vi "IMAQdx Acquisition Template (Host).vi"() -> ()   [LabVIEW 2016]
uses:
  <vilib>/userdefined/High Color/IMAQdx.ctl
  <vilib>/vision/driver/IMAQdx.llb/IMAQdx Acquisition Mode.ctl
  <vilib>/vision/driver/IMAQdx.llb/IMAQdx Buffer Number Mode.ctl
  <vilib>/FPGAPlugInAG/roboRIO/niLvFpga_Open_roboRIO.vi
  <vilib>/rvi/interface/common/dynamic/niFpgaDynamicAddResources.vi
  <vilib>/FPGAPlugInAG/Dynamic/niLvFpga_Download_Dynamic.vi
  <vilib>/FPGAPlugInAG/Dynamic/niLvFpga_Run_Dynamic.vi
  <vilib>/visionFPGA/Basics/Configure Image Transfer to Target/IMAQ FPGA Configure Image Transfer to Target U32.vi
  <vilib>/Utility/error.llb/Error Cluster From Error Code.vi
  <vilib>/rvi/errors/niLvFpgaAdjustHostInterfaceError.vi
  <vilib>/visionFPGA/Basics/Image Transfer to Target/IMAQ FPGA Image Transfer to Target U32.vi
  <vilib>/rvi/interface/common/niFpgaWaitOnOcc.vi
  <vilib>/FPGAPlugInAG/Dynamic/niLvFpga_Close_Dynamic.vi
  <vilib>/rvi/interface/nirviOpenFPGA/nirviOpenFPGA.xnode
  FPGA Bitfiles/ImageProcessingw_FPGATarget2_ImageProcessingw_ZcF2hsHpmf8.lvbitx
  Image Processing with Vision Assistant (FPGA).vi
  <vilib>/rvi/interface/nirviMethod/nirviMethod.xnode
  <vilib>/rvi/interface/nirviReadWriteControl/nirviReadWriteControl.xnode
  <vilib>/rvi/interface/nirviCloseFPGA/nirviCloseFPGA.xnode
  <vilib>/vision/driver/NI_Vision_Acquisition_Software.lvlib
  <resource>/objmgr/imaqdx.rc
  <vilib>/visionFPGA/NI_VDM_FPGA_Basics.lvlib
  <vilib>/rvi/interface/Simulation/niFpgaSimulationCallBeginRW.vi
  <vilib>/rvi/errors/niLvFpgaMergeErrorWithErrorCode.vi
  <vilib>/FPGAPlugInAG/Dynamic/niLvFpga_ReadFifo_Dynamic.vi
  <vilib>/FPGAPlugInAG/Dynamic/niLvFpga_ConfigureFifo_Dynamic.vi
  <vilib>/FPGAPlugInAG/Dynamic/niLvFpga_StartFifo_Dynamic.vi
  NiFpgaLv.dll
panel:
  out "OriImage Err out":errorcluster
  out "Image":T1(plugin-control)
  out "Count":i32
  out "error out 2":errorcluster
  out "sendPic":bool=TRUE
  in  "Camera":T2
  out "Error Out":errorcluster
  in  "Stop":bool
  # "Overview: Demonstrates how to acquire an image from a camera using the IMAQdx API, transfer the image to a FPGA target for processing, and retrieve the processed image for display or further processing on the host.\nRequirements:\n- LabVIEW FPGA\n- Vision Acquisition Software\n- Vision Development Module\nInstructions:\n1. Select a Camera\n2. Run the VI."
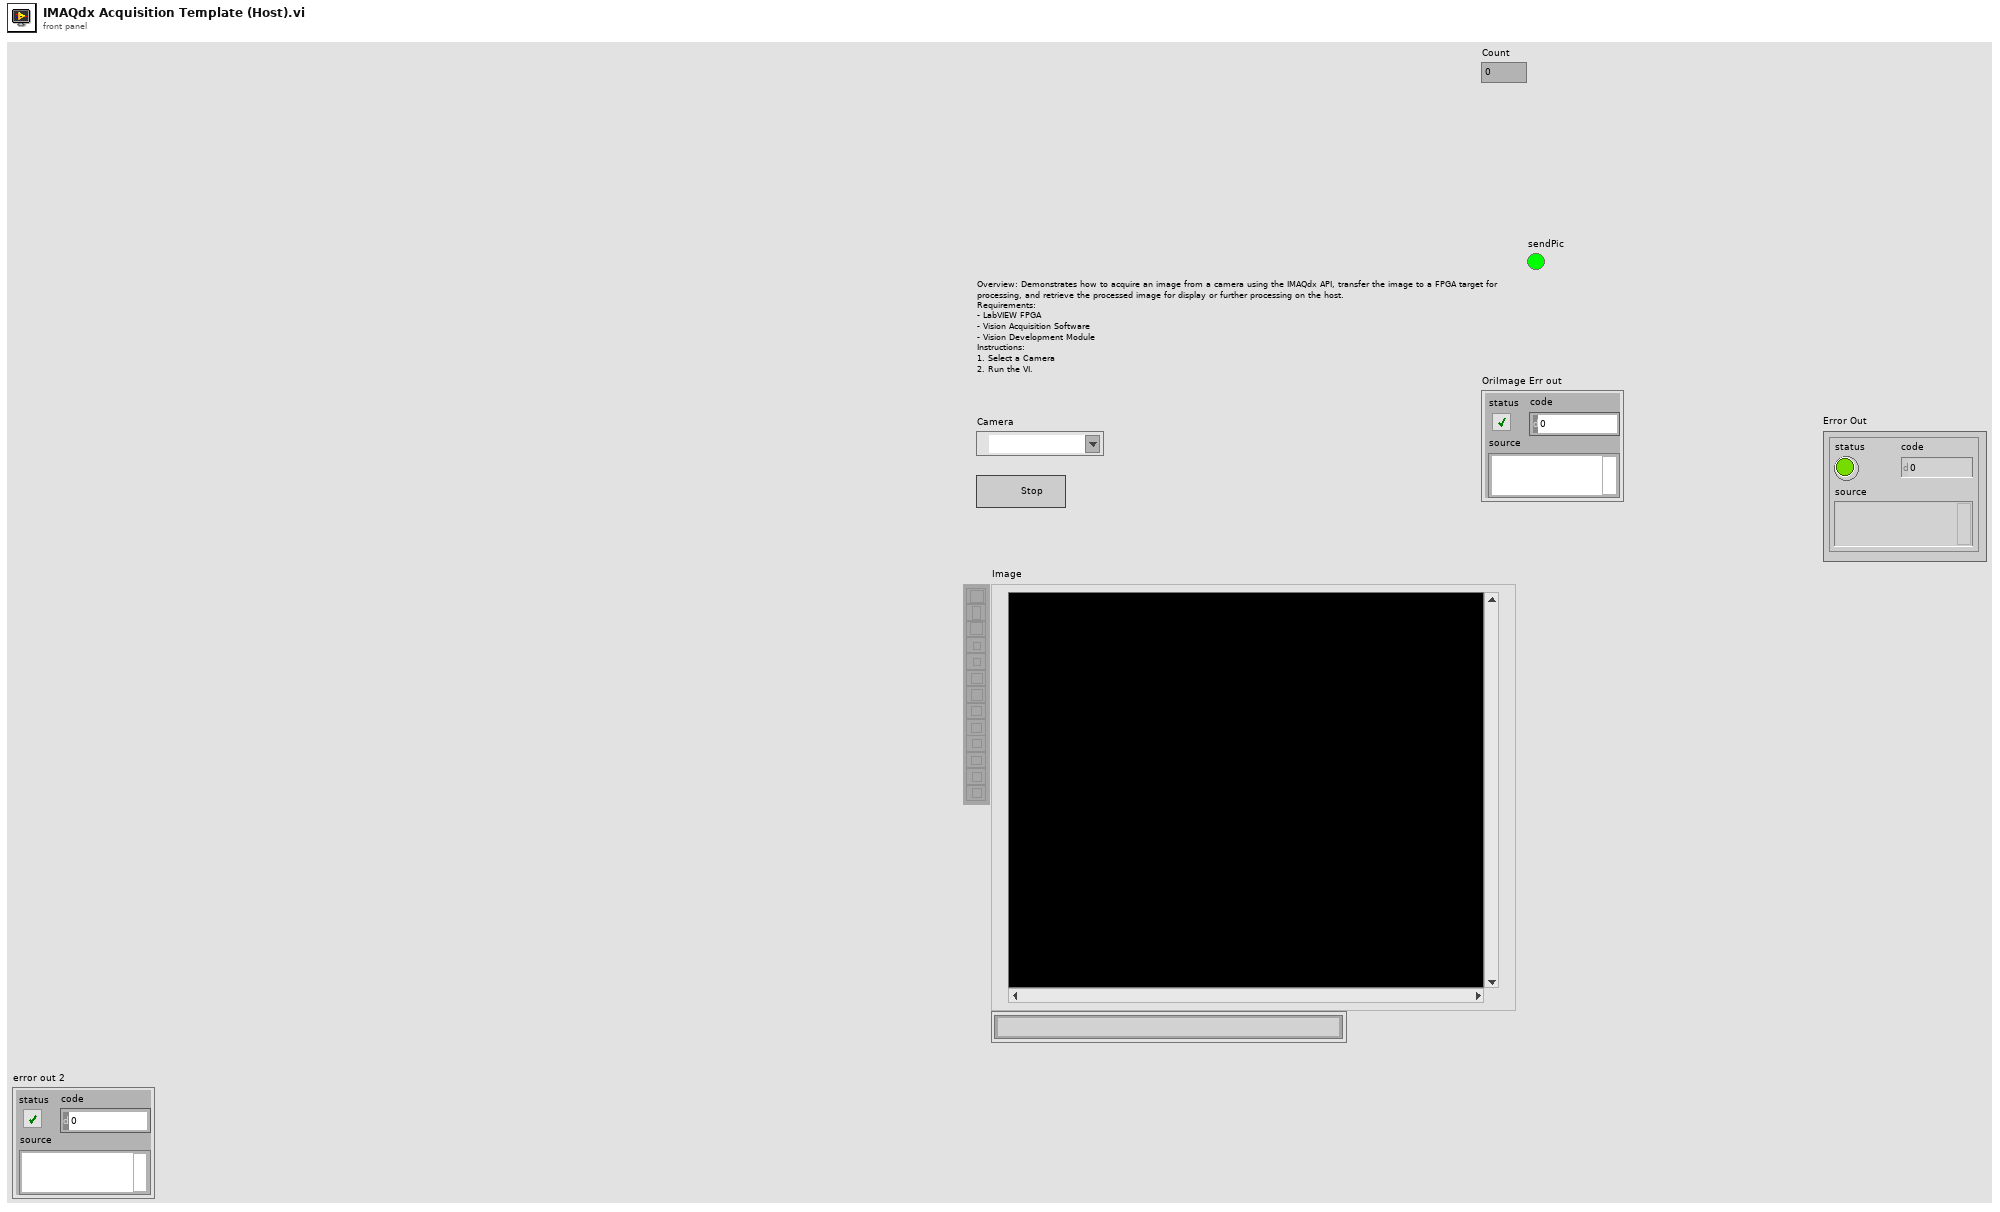
[diagram p1: front panel]
types:
  T1 = typedef "IMAQ Image.ctl" = refnum<image>
  T2 = typedef "IMAQdx.ctl" = refnum<k21>
  T3 = typedef "Image Type" = u32
  T4 = typedef "NI_Vision_Acquisition_Software.lvlib/IMAQdx Acquisition Mode.ctl" = enum32{"One Shot", "Continuous"}
  T5 = typedef "NI_Vision_Acquisition_Software.lvlib/IMAQdx Buffer Number Mode.ctl" = enum32{"Next", "Last", "Buffer Number", "Every", "Last New"}
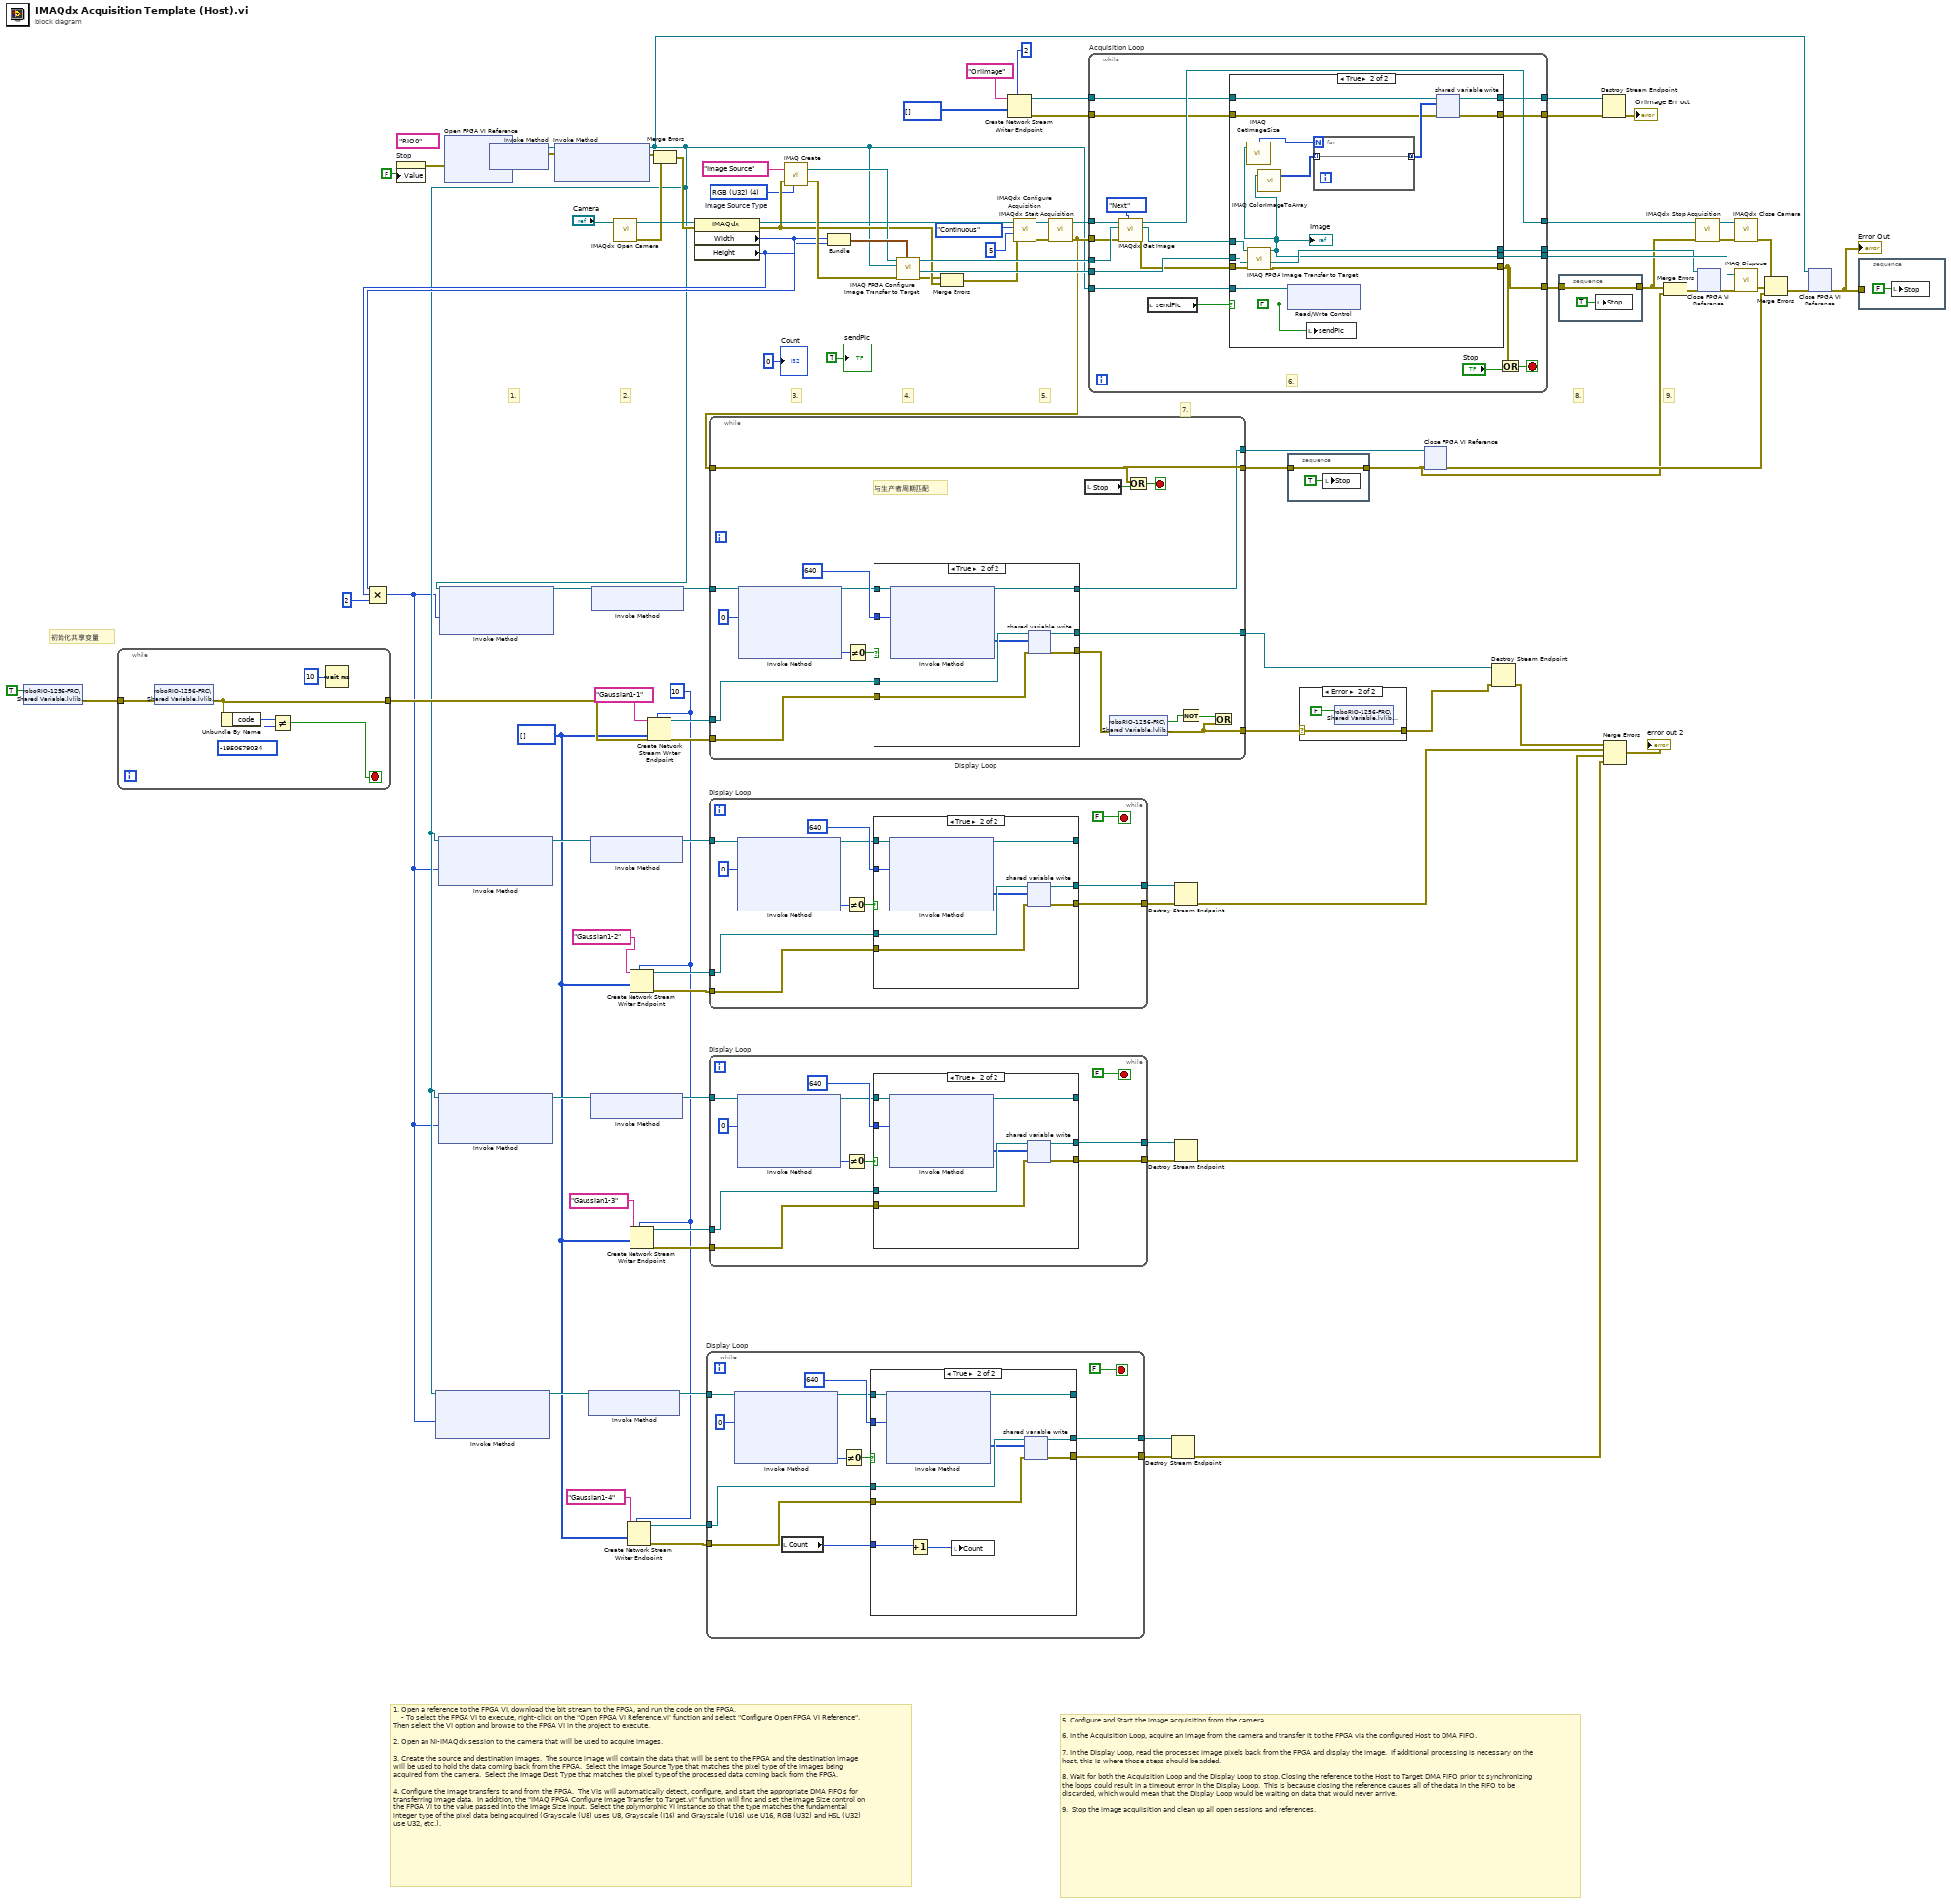
[diagram p0: block diagram]
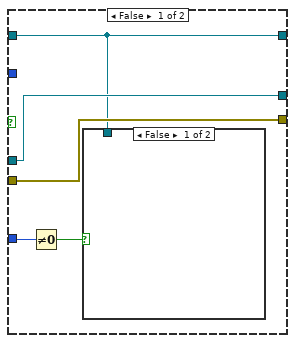
[diagram p2: hidden frame]
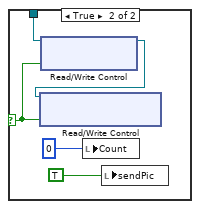
[diagram p3: hidden frame]
diagram:
  w4 = i32[] []
  w5 = 10 ("writer buffer size")
  w63 = T3 4 items=["Grayscale (U8)", "Grayscale (I16)", "Grayscale (SGL)", "Complex (CSG)", "RGB (U32)", "HSL (U32)", "RGB (U64)", "Grayscale (U16)"]  # Image Source Type
  # "初始化共享变量"
  # "5. Configure and Start the image acquisition from the camera.\n\n6. In the Acquisition Loop, acquire an image from the camera and transfer it to the FPGA via the configured Host to DMA FIFO.\n\n7. In the Display Loop, read the processed image pixels back from the FPGA and display the image.  If additional processing is necessary on the host, this is where those steps should be added.\n\n8. Wait for both the Acquisition Loop and the Display Loop to stop. Closing the reference to the Host to Target DMA FIFO prior to synchronizing the loops could result in a timeout error in the Display Loop.  This is because closing the reference causes all of the data in the FIFO to be discarded, which would mean that the Display Loop would be waiting on data that would never arrive.\n\n9.  Stop the image acquiisition and clean up all open sessions and references."
  # "1. Open a reference to the FPGA VI, download the bit stream to the FPGA, and run the code on the FPGA.\n    - To select the FPGA VI to execute, right-click on the \"Open FPGA VI Reference.vi\" function and select \"Configure Open FPGA VI Reference\".  Then select the VI option and browse to the FPGA VI in the project to execute.\n\n2. Open an NI-IMAQdx session to the camera that will be used to acquire images.\n\n3. Create the source and destination images.  The source image will contain the data that will be sent to the FPGA and the destination image will be used to hold the data coming back from the FPGA.  Select the Image Source Type that matches the pixel type of the images being acquired from the camera.  Select the Image Dest Type that matches the pixel type of the processed data coming back from the FPGA.\n\n4. Configure the image transfers to and from the FPGA.  The VIs will automatically detect, configure, and start the appropriate DMA FIFOs for transferring image data.  In addition, the \"IMAQ FPGA Configure Image Transfer to Target.vi\" function will find and set the Image Size control on the FPGA VI to the value passed in to the Image Size input.  Select the polymorphic VI instance so that the type matches the fundamental integer type of the pixel data being acquired (Grayscale (U8) uses U8, Grayscale (I16) and Grayscale (U16) use U16, RGB (U32) and HSL (U32) use U32, etc.)."
  # "9."
  # "8."
  # "7."
  # "6."
  # "5."
  # "4."
  # "3."
  # "2."
  # "1."
  n1 = shared-variable "roboRIO-1256-FRC\\Shared Variable.lvlib\\Active"(TRUE ("Active?")) -> (error out=w49:errorcluster)  [unwired: 1 in]
  n2 = while {
    tunnel: w49 -> [w106]
    tunnel: [w103] -> w48
    stop <- w102 stop-if-true
    n3 = shared-variable "roboRIO-1256-FRC\\Shared Variable.lvlib\\Active"(error in=w106) -> (error out=w103:errorcluster)  [unwired: 1 out]
    n4 = Unbundle By Name(w103) -> ("code"=w105:i32)
    n5 = Not Equal?(x=w105, y=-1950679034) -> (x != y?=w102:bool)
    n6 = Wait (ms)(milliseconds to wait=u32 10) -> ()  [unwired: 1 out]
  }
  n7 = property on="Stop" class="Bool (strict)"("Value"=FALSE ("Stop")) -> (error out=w98:errorcluster)  [unwired: 2 in, 1 out]
  n8 = xnode "Open FPGA VI Reference"("error in"=w98, "resource name"=tag "RIO0") -> ("FPGA VI Reference Out"=w94:refnum<k20>, "error out"=w95:errorcluster)
  n9 = xnode "Invoke Method"("FPGA VI Reference In"=w94, "error in"=w95) -> ("FPGA VI Reference Out"=w97:refnum<k20>, "error out"=w96:errorcluster)
  n10 = xnode "Invoke Method"("FPGA VI Reference In"=w97, "error in"=w96) -> ("FPGA VI Reference Out"=w3:refnum<k20>, "error out"=w83:errorcluster)  [unwired: 1 in]
  n11 = call <vilib>:"IMAQdx Open Camera.vi"("Session In"="Camera") -> ("error out"=w68:errorcluster, "Session Out"=w69:T2)  [unwired: 9 in]
  n12 = Create Network Stream Writer Endpoint(7:w5, 9:w4, 11:"Gaussian1-4" ("writer name")) -> (0:w8:errorcluster, 3:w9:refnum<k21>)  [unwired: 4 in]
  n13 = Create Network Stream Writer Endpoint(7:w5, 9:w4, 11:"Gaussian1-2" ("writer name")) -> (0:w23:errorcluster, 3:w24:refnum<k21>)  [unwired: 4 in]
  n14 = Create Network Stream Writer Endpoint(7:w5, 9:w4, 11:"Gaussian1-3" ("writer name")) -> (0:w18:errorcluster, 3:w17:refnum<k21>)  [unwired: 4 in]
  n15 = Create Network Stream Writer Endpoint(7:w5, 8:w48, 9:w4, 11:"Gaussian1-1" ("writer name")) -> (0:w44:errorcluster, 3:w43:refnum<k21>)  [unwired: 3 in]
  n16 = Merge Errors(w83, w68) -> (w67:errorcluster)
  n17 = property class="IMAQdx"(reference=w69, error in=w67) -> (reference out=w76:T2, error out=w64:errorcluster, "Width"=w42:u32, "Height"=w41:u32)
  n18 = Compound Arithmetic op=MULTIPLY(w42, w41, u32 2 ("value")) -> (w2:u32)
  n19 = xnode "Invoke Method"("FPGA VI Reference In"=w3, "Requested Depth"=w2) -> ("FPGA VI Reference Out"=w7:refnum<k20>)  [unwired: 1 in, 2 out]
  n20 = xnode "Invoke Method"("FPGA VI Reference In"=w3, "Requested Depth"=w2) -> ("FPGA VI Reference Out"=w22:refnum<k20>)  [unwired: 1 in, 2 out]
  n21 = xnode "Invoke Method"("FPGA VI Reference In"=w3, "Requested Depth"=w2) -> ("FPGA VI Reference Out"=w19:refnum<k20>)  [unwired: 1 in, 2 out]
  n22 = xnode "Invoke Method"("FPGA VI Reference In"=w3, "Requested Depth"=w2) -> ("FPGA VI Reference Out"=w53:refnum<k20>)  [unwired: 1 in, 2 out]
  n23 = xnode "Invoke Method"("FPGA VI Reference In"=w7) -> ("FPGA VI Reference Out"=w6:refnum<k20>)  [unwired: 1 in, 1 out]
  n24 = xnode "Invoke Method"("FPGA VI Reference In"=w22) -> ("FPGA VI Reference Out"=w21:refnum<k20>)  [unwired: 1 in, 1 out]
  n25 = xnode "Invoke Method"("FPGA VI Reference In"=w19) -> ("FPGA VI Reference Out"=w20:refnum<k20>)  [unwired: 1 in, 1 out]
  n26 = xnode "Invoke Method"("FPGA VI Reference In"=w53) -> ("FPGA VI Reference Out"=w52:refnum<k20>)  [unwired: 1 in, 1 out]
  n27 = while "Display Loop" {
    tunnel: [w118] -> w12
    tunnel: w8 -> [w117]
    tunnel: w9 -> [w116]
    tunnel: [w108] -> w11
    tunnel: w6 -> [w107]
    stop <- FALSE stop-if-true
    (unwired) u32 640 ("Number of Elements")
    n28 = xnode "Invoke Method"("FPGA VI Reference In"=w107, "Number of Elements"=u32 0) -> ("FPGA VI Reference Out"=w110:refnum<k20>, "Elements Remaining"=w111:u32)  [unwired: 2 in, 2 out]
    n29 = local read "Count"() -> (w112:i32)
    n30 = Not Equal To 0?(x=w111) -> (x != 0?=w115:bool)
    n31 = case shown="True" w115 {
      tunnel: w110 -> [w119 w138]
      tunnel: [w123 w137] -> w118
      tunnel: w117 -> [w122 w136]
      tunnel: w116 -> [w123 w135]
      tunnel: [w122 w134] -> w108
      tunnel: [w119 w132] -> _
      tunnel: 640 -> [_ w131]
      tunnel: w112 -> [w121 w130]
      frame False {
        n32 = Not Equal To 0?(x=w121) -> (x != 0?=w120:bool)
        n33 = case shown="False" w120 {
          selector: w120 -> [_ w125]
          tunnel: w119 -> [_ w128]
          frame False {
          }
          frame True {
            n34 = xnode "Read/Write Control"("FPGA VI Reference In"=w128, "StartOfImage"=w125) -> ("FPGA VI Reference Out"=w127:refnum<k20>)  [unwired: 1 in, 1 out]
            n35 = xnode "Read/Write Control"("FPGA VI Reference In"=w127, "Ready For Output"=w125) -> ()  [unwired: 1 in, 2 out]
            n36 = local write "Count"(0) -> ()
            n37 = local write "sendPic"(TRUE ("start")) -> ()
          }
        }
      }
      frame True {
        n38 = xnode "Invoke Method"("FPGA VI Reference In"=w138, "Number of Elements"=w131) -> ("FPGA VI Reference Out"=w132:refnum<k20>, "Data"=w133:u8[])  [unwired: 2 in, 2 out]
        n39 = Increment(x=w130) -> (x+1=w129:i32)
        n40 = local write "Count"(w129) -> ()
        n41 = shared-variable-write(w135, w136, w133) -> (w137:refnum<k21>, w134:errorcluster)  [unwired: 1 in, 1 out]
      }
    }
  }
  n42 = while "Display Loop" {
    tunnel: [w149] -> w31
    tunnel: w23 -> [w148]
    tunnel: w24 -> [w147]
    tunnel: [w140] -> w30
    tunnel: w21 -> [w139]
    stop <- FALSE stop-if-true
    (unwired) u32 640 ("Number of Elements")
    n43 = xnode "Invoke Method"("FPGA VI Reference In"=w139, "Number of Elements"=u32 0) -> ("FPGA VI Reference Out"=w142:refnum<k20>, "Elements Remaining"=w143:u32)  [unwired: 2 in, 2 out]
    n44 = Not Equal To 0?(x=w143) -> (x != 0?=w146:bool)
    n45 = case shown="True" w146 {
      tunnel: w142 -> [w150 w160]
      tunnel: [w152 w159] -> w149
      tunnel: w148 -> [w151 w158]
      tunnel: w147 -> [w152 w157]
      tunnel: [w151 w156] -> w140
      tunnel: [w150 w154] -> _
      tunnel: 640 -> [_ w153]
      frame False {
      }
      frame True {
        n46 = xnode "Invoke Method"("FPGA VI Reference In"=w160, "Number of Elements"=w153) -> ("FPGA VI Reference Out"=w154:refnum<k20>, "Data"=w155:u8[])  [unwired: 2 in, 2 out]
        n47 = shared-variable-write(w157, w158, w155) -> (w159:refnum<k21>, w156:errorcluster)  [unwired: 1 in, 1 out]
      }
    }
  }
  n48 = while "Display Loop" {
    tunnel: [w171] -> w14
    tunnel: w18 -> [w170]
    tunnel: w17 -> [w169]
    tunnel: [w162] -> w15
    tunnel: w20 -> [w161]
    stop <- FALSE stop-if-true
    (unwired) u32 640 ("Number of Elements")
    n49 = xnode "Invoke Method"("FPGA VI Reference In"=w161, "Number of Elements"=u32 0) -> ("FPGA VI Reference Out"=w164:refnum<k20>, "Elements Remaining"=w165:u32)  [unwired: 2 in, 2 out]
    n50 = Not Equal To 0?(x=w165) -> (x != 0?=w168:bool)
    n51 = case shown="True" w168 {
      tunnel: w164 -> [w172 w182]
      tunnel: [w174 w181] -> w171
      tunnel: w170 -> [w173 w180]
      tunnel: w169 -> [w174 w179]
      tunnel: [w173 w178] -> w162
      tunnel: [w172 w176] -> _
      tunnel: 640 -> [_ w175]
      frame False {
      }
      frame True {
        n52 = xnode "Invoke Method"("FPGA VI Reference In"=w182, "Number of Elements"=w175) -> ("FPGA VI Reference Out"=w176:refnum<k20>, "Data"=w177:u8[])  [unwired: 2 in, 2 out]
        n53 = shared-variable-write(w179, w180, w177) -> (w181:refnum<k21>, w178:errorcluster)  [unwired: 1 in, 1 out]
      }
    }
  }
  n54 = call "IMAQ Create"("Image Name"="Image Source", "Image Type"=w63, "error in (no error)"=w64) -> ("New Image"=w74:T1, "error out"=w82:errorcluster)  [unwired: 2 in]
  n55 = Bundle("Width"=w42, "Height"=w41) -> (w81:cluster{"Width":u32, "Height":u32})  [unwired: 1 in]
  n56 = call-poly <vilib>:"IMAQ FPGA Configure Image Transfer to Target.vi"("Image Size"=w81, "error in (no error)"=w82, "FPGA VI Reference In"=w3, "Image"=w74) -> ("error out"=w57:errorcluster, "DMA FIFO Reference Out"=w92:refnum<k20>, "Image Out"=w93:T1)  [unwired: 4 in, 1 out]
  n57 = Merge Errors(w57, w64) -> (w56:errorcluster)
  n58 = Create Network Stream Writer Endpoint(7:2 ("writer buffer size"), 9:i32[] [], 11:"OriImage" ("writer name")) -> (0:w35:errorcluster, 3:w36:refnum<k21>)  [unwired: 4 in]
  n59 = call <vilib>:"IMAQdx Configure Acquisition.vi"("error in"=w56, "Number of Buffers"=u32 5, "Continuous?"=IMAQdx_Acquisition_Mode."Continuous", "Session In"=w76) -> ("error out"=w79:errorcluster, "Session Out"=w80:T2)  [unwired: 6 in]
  n60 = call <vilib>:"IMAQdx Start Acquisition.vi"("error in"=w79, "Session In"=w80) -> ("error out"=w55:errorcluster, "Session Out"=w75:T2)  [unwired: 8 in]
  n61 = while "Display Loop" {
    tunnel: w55 -> [w198]
    tunnel: [w186] -> w89
    tunnel: [w198] -> w88
    tunnel: w52 -> [w187]
    tunnel: [w196] -> w46
    tunnel: [w195] -> w45
    tunnel: w44 -> [w194]
    tunnel: w43 -> [w193]
    stop <- w199 stop-if-true
    (unwired) u32 640 ("Number of Elements")
    # "与生产者周期匹配"
    n62 = xnode "Invoke Method"("FPGA VI Reference In"=w187, "Number of Elements"=u32 0) -> ("FPGA VI Reference Out"=w183:refnum<k20>, "Elements Remaining"=w184:u32)  [unwired: 2 in, 2 out]
    n63 = Not Equal To 0?(x=w184) -> (x != 0?=w189:bool)
    n64 = case shown="True" w189 {
      tunnel: w183 -> [w200 w210]
      tunnel: [w202 w209] -> w195
      tunnel: w194 -> [w201 w208]
      tunnel: w193 -> [w202 w207]
      tunnel: [w201 w206] -> w192
      tunnel: [w200 w204] -> w186
      tunnel: 640 -> [_ w203]
      frame False {
      }
      frame True {
        n65 = xnode "Invoke Method"("FPGA VI Reference In"=w210, "Number of Elements"=w203) -> ("FPGA VI Reference Out"=w204:refnum<k20>, "Data"=w205:u8[])  [unwired: 2 in, 2 out]
        n66 = shared-variable-write(w207, w208, w205) -> (w209:refnum<k21>, w206:errorcluster)  [unwired: 1 in, 1 out]
      }
    }
    n67 = local read "Stop"() -> (w197:bool)
    n68 = shared-variable "roboRIO-1256-FRC\\Shared Variable.lvlib\\Active"(error in=w192) -> (w190:bool, error out=w196:errorcluster)
    n69 = Or(x=w198, y=w197) -> (x .or. y?=w199:bool)
    n70 = Not(x=w190) -> (.not. x?=w191:bool)
    n71 = Or(x=w191, y=w196) -> ()  [unwired: 1 out]
  }
  n72 = while "Acquisition Loop" {
    tunnel: [w220] -> w61
    tunnel: w93 -> [w225]
    tunnel: w92 -> [w222]
    tunnel: [w221] -> w62
    tunnel: [w218] -> w91
    tunnel: w75 -> [w226]
    tunnel: [w224] -> w71
    tunnel: w55 -> [w223]
    tunnel: w3 -> [w216]
    tunnel: w36 -> [w214]
    tunnel: w35 -> [w213]
    tunnel: [w212] -> w34
    tunnel: [w211] -> w33
    stop <- w228 stop-if-true
    n73 = call <vilib>:"IMAQdx Get Image.vi"("Buffer Number Mode (Next)"=IMAQdx_Buffer_Number_Mode."Next", "error in"=w223, "Image In"=w225, "Session In"=w226) -> ("error out"=w217:errorcluster, "Image Out"=w219:T1, "Session Out"=w224:T2)  [unwired: 4 in, 1 out]
    n74 = local read "sendPic"() -> (w215:bool)
    n75 = case shown="True" w215 {
      tunnel: w222 -> [w234 w249]
      tunnel: [w234 w245] -> w221
      tunnel: [w233 w246] -> w220
      tunnel: w219 -> [w232 w248]
      tunnel: [w232 w240] -> w218
      tunnel: w217 -> [w233 w247]
      tunnel: w216 -> [_ w243]
      tunnel: w214 -> [w231 w238]
      tunnel: w213 -> [w230 w237]
      tunnel: [w231 w236] -> w212
      tunnel: [w230 w235] -> w211
      frame False {
      }
      frame True {
        w244 = FALSE ("EndOfImage")
        n76 = call-poly <vilib>:"IMAQ FPGA Image Transfer to Target.vi"("error in (no error)"=w247, "DMA FIFO Reference In"=w249, "Image"=w248) -> ("error out"=w246:errorcluster, "DMA FIFO Reference Out"=w245:refnum<k20>, "Image Out"=w240:T1)  [unwired: 6 in]
        "Image" <- w240
        n77 = call "IMAQ GetImageSize"("Image"=w240) -> ("X Resolution"=w242:i32)  [unwired: 3 in, 2 out]
        n78 = call "IMAQ ColorImageToArray"("Image"=w240) -> ("Image Pixels (U32)"=w241:u32[][])  [unwired: 3 in, 2 out]
        n79 = xnode "Read/Write Control"("FPGA VI Reference In"=w243, "StartOfImage"=w244) -> ()  [unwired: 1 in, 2 out]
        n80 = local write "sendPic"(w244) -> ()
        n81 = for {
          N: w242 -> [_]
          tunnel: w241 -> [w250] mode=indexing
          tunnel: [w250] -> w239 mode=concatenating
        }
        n82 = shared-variable-write(w238, w237, w239) -> (w236:refnum<k21>, w235:errorcluster)  [unwired: 1 in, 1 out]
      }
    }
    n83 = Or(x=w220, y="Stop") -> (x .or. y?=w228:bool)
  }
  n84 = Destroy Stream Endpoint(8:w11, 11:w12) -> (0:w1:errorcluster)
  n85 = Destroy Stream Endpoint(8:w30, 11:w31) -> (0:w26:errorcluster)
  n86 = Destroy Stream Endpoint(8:w15, 11:w14) -> (0:w13:errorcluster)
  n87 = stacked-sequence {
    tunnel: w88 -> [w251]
    tunnel: [w251] -> w60
    frame #0 {
      n88 = local write "Stop"(TRUE ("Stop")) -> ()
    }
  }
  n89 = case shown="Error" w46 {
    selector: w46 -> [w253 w254]
    tunnel: [w253 w254] -> w29
    frame No Error {
    }
    frame Error {
      n90 = shared-variable "roboRIO-1256-FRC\\Shared Variable.lvlib\\Active"(FALSE ("Active?")) -> ()  [unwired: 1 in, 1 out]
    }
  }
  n91 = xnode "Close FPGA VI Reference"("FPGA VI Reference In"=w89, "error in"=w60) -> ("error out"=w87:errorcluster)
  n92 = Destroy Stream Endpoint(8:w29, 11:w45) -> (0:w27:errorcluster)
  n93 = stacked-sequence {
    tunnel: w61 -> [w256]
    tunnel: [w256] -> w58
    frame #0 {
      n94 = local write "Stop"(TRUE ("Stop")) -> ()
    }
  }
  n95 = Destroy Stream Endpoint(8:w33, 11:w34) -> (0:→"OriImage Err out":errorcluster)
  n96 = Merge Errors(w27, w26, w13, w1) -> (→"error out 2":errorcluster)
  n97 = Merge Errors(w58, w60) -> (w59:errorcluster)
  n98 = call <vilib>:"IMAQdx Stop Acquisition.vi"("error in"=w58, "Session In"=w71) -> ("error out"=w72:errorcluster, "Session Out"=w73:T2)  [unwired: 8 in]
  n99 = xnode "Close FPGA VI Reference"("FPGA VI Reference In"=w62, "error in"=w59) -> ("error out"=w90:errorcluster)
  n100 = call <vilib>:"IMAQdx Close Camera.vi"("error in"=w72, "Session In"=w73) -> ("error out"=w70:errorcluster)  [unwired: 9 in]
  n101 = call "IMAQ Dispose"("Image"=w91, "error in (no error)"=w90) -> ("error out"=w86:errorcluster)  [unwired: 4 in]
  n102 = Merge Errors(w70, w86, w87) -> (w66:errorcluster)
  n103 = xnode "Close FPGA VI Reference"("FPGA VI Reference In"=w3, "error in"=w66) -> ("error out"=w65:errorcluster)
  "Error Out" <- w65
  n104 = stacked-sequence {
    tunnel: w65 -> [_]
    frame #0 {
      n105 = local write "Stop"(FALSE ("Stop")) -> ()
    }
  }
  "sendPic" <- TRUE
  "Count" <- 0
